vi "Simulation-01.vi"() -> (0 "lib error out":errorcluster, 3 "success":bool)   [LabVIEW 2020]
uses:
  librarian_class/librarian.lvclass
  client_class/client.lvclass
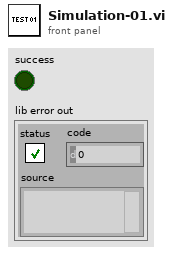
[diagram p1: front panel]
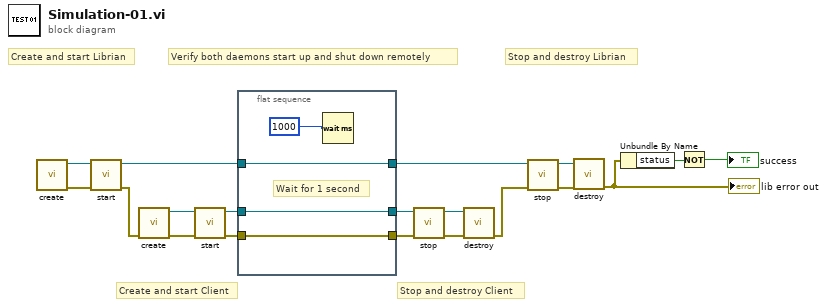
[diagram p0: block diagram]
diagram:
  # "Verify both daemons start up and shut down remotely"
  # "Stop and destroy Librian"
  # "Stop and destroy Client"
  # "Create and start Client"
  # "Create and start Librian"
  n1 = call "create.vi"() -> ("error out"=w18:errorcluster, "librarian_sm out"=w19:refnum<class "librarian.lvclass">)  [unwired: 10 in]
  n2 = call "start.vi"("error in (no error)"=w18, "librarian_sm in"=w19) -> ("error out"=w11:errorcluster, "librarian_sm out"=w8:refnum<class "librarian.lvclass">)  [unwired: 8 in]
  n3 = call "create.vi"("error in (no error)"=w11) -> ("error out"=w14:errorcluster, "librarian_sm out"=w15:refnum<class "client.lvclass">)  [unwired: 9 in]
  n4 = call "start.vi"("error in (no error)"=w14, "librarian_sm in"=w15) -> ("error out"=w10:errorcluster, "librarian_sm out"=w9:refnum<class "client.lvclass">)  [unwired: 8 in]
  n5 = flat-sequence {
    tunnel: w10 -> [w21]
    tunnel: w9 -> [w20]
    tunnel: w8 -> [w22]
    tunnel: [w22] -> w7
    tunnel: [w21] -> w6
    tunnel: [w20] -> w5
    frame #0 {
      # "Wait for 1 second"
      n6 = Wait (ms)(milliseconds to wait=u32 1000) -> ()  [unwired: 1 out]
    }
  }
  n7 = call "stop.vi"("error in (no error)"=w6, "librarian_sm in"=w5) -> ("error out"=w12:errorcluster, "librarian_sm out"=w13:refnum<class "client.lvclass">)  [unwired: 8 in]
  n8 = call "destroy.vi"("error in (no error)"=w12, "librarian_sm in"=w13) -> ("error out"=w4:errorcluster)  [unwired: 8 in, 1 out]
  n9 = call "stop.vi"("error in (no error)"=w4, "librarian_sm in"=w7) -> ("error out"=w16:errorcluster, "librarian_sm out"=w17:refnum<class "librarian.lvclass">)  [unwired: 8 in]
  n10 = call "destroy.vi"("error in (no error)"=w16, "librarian_sm in"=w17) -> ("error out"=w3:errorcluster)  [unwired: 8 in, 1 out]
  "lib error out" <- w3
  n11 = Unbundle By Name(w3) -> ("status"=w2:bool)
  n12 = Not(x=w2) -> (.not. x?=→"success":bool)
